vi "Check Conditions.vi"(7 "Reset":bool, 9 "Dist":dbl, 11 "Condition":i32) -> (3 "Done?":bool)   [LabVIEW 2014]
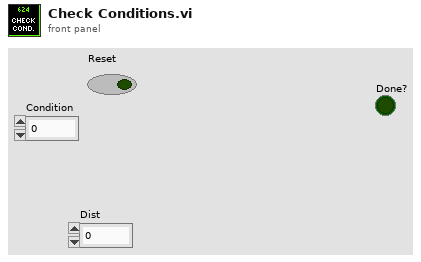
[diagram p1: front panel]
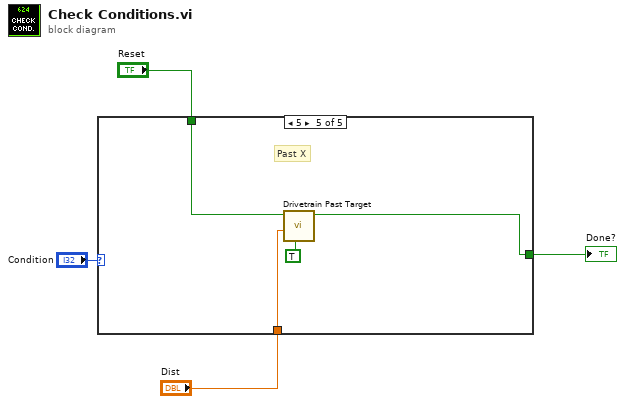
[diagram p0: block diagram]
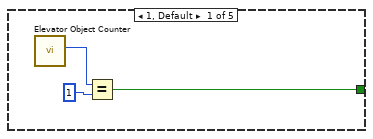
[diagram p2: hidden frame]
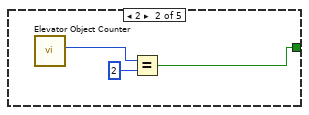
[diagram p3: hidden frame]
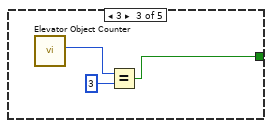
[diagram p4: hidden frame]
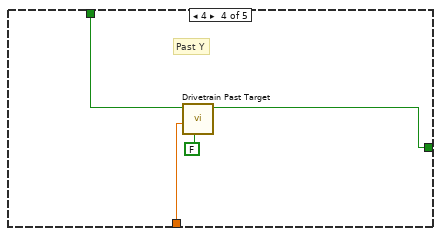
[diagram p5: hidden frame]
diagram:
  n1 = case shown="5" "Condition" {
    tunnel: [w5 w8 w11 w17 w21] -> w3
    tunnel: "Reset" -> [_ _ _ w16 w20]
    tunnel: "Dist" -> [_ _ _ w14 w18]
    frame 1, Default {
      n2 = call "Elevator Object Counter.vi"() -> ("Tote Count"=w7:i8)  [unwired: 10 in, 1 out]
      n3 = Equal?(x=w7, y=i8 1) -> (x = y?=w5:bool)
    }
    frame 2 {
      n4 = call "Elevator Object Counter.vi"() -> ("Tote Count"=w9:i8)  [unwired: 10 in, 1 out]
      n5 = Equal?(x=w9, y=i8 2) -> (x = y?=w8:bool)
    }
    frame 3 {
      n6 = call "Elevator Object Counter.vi"() -> ("Tote Count"=w12:i8)  [unwired: 10 in, 1 out]
      n7 = Equal?(x=w12, y=i8 3) -> (x = y?=w11:bool)
    }
    frame 4 {
      # "Past Y"
      n8 = call "Drivetrain Past Target.vi"("Use X Distance?"=FALSE, "Distance Target"=w14, "Reset"=w16) -> ("Past Target?"=w17:bool)  [unwired: 8 in]
    }
    frame 5 {
      # "Past X"
      n9 = call "Drivetrain Past Target.vi"("Use X Distance?"=TRUE, "Distance Target"=w18, "Reset"=w20) -> ("Past Target?"=w21:bool)  [unwired: 8 in]
    }
  }
  "Done?" <- w3
